vi "HoldOrRelease.vi"(10 "Delay":dbl, 11 "Right Bumper":bool) -> (2 "Call Auto-Hatch":bool, 3 "Call Toggle":bool)   [LabVIEW 2018]
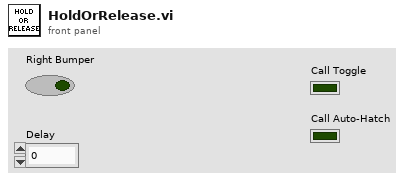
[diagram p1: front panel]
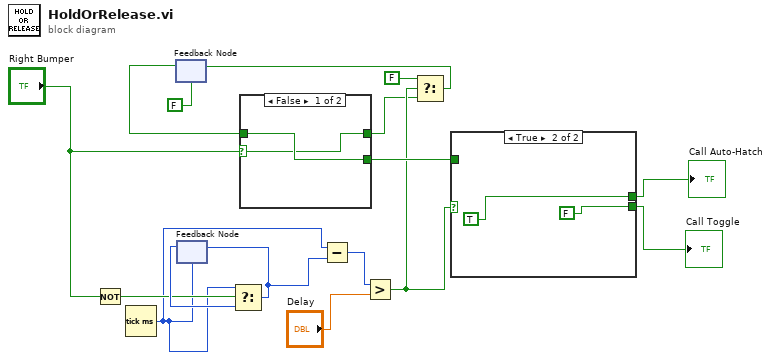
[diagram p0: block diagram]
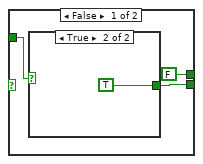
[diagram p2: hidden frame]
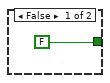
[diagram p3: hidden frame]
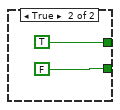
[diagram p4: hidden frame]
diagram:
  n1 = Not(x="Right Bumper") -> (.not. x?=w11:bool)
  n2 = Tick Count (ms)() -> (millisecond timer value=w5:u32)
  n3 = feedback #1(FALSE) -> (w12:bool)
  n4 = feedback #2(w5) -> (w16:u32)
  n5 = Select(t=w5, s=w11, f=w16) -> (s? t:f=w14:u32)
  n6 = feedback-in #2(w14) -> ()
  n7 = case shown="False" "Right Bumper" {
    selector: "Right Bumper" -> [w17 _]
    tunnel: w12 -> [w18 _]
    tunnel: [w17 TRUE] -> w8
    tunnel: [w18 FALSE] -> w10
    frame False {
    }
    frame True {
    }
  }
  n8 = Subtract(x=w5, y=w14) -> (x-y=w13:u32)
  n9 = Greater?(x=w13, y="Delay") -> (0:w9:bool)
  n10 = Select(t=FALSE, s=w9, f=w8) -> (s? t:f=w6:bool)
  n11 = feedback-in #1(w6) -> ()
  n12 = case shown="True" w9 {
    tunnel: w10 -> [w23 _]
    tunnel: [FALSE TRUE ("Call AutoHatch")] -> w1
    tunnel: [w22 FALSE] -> w2
    frame False {
      n13 = case shown="True" w23 {
        tunnel: [FALSE TRUE ("Call Toggle")] -> w22
        frame False {
        }
        frame True {
        }
      }
    }
    frame True {
    }
  }
  "Call Toggle" <- w2
  "Call Auto-Hatch" <- w1
